vi "Simulated Starter Kit 2.0 Roaming.vi"() -> ()   [LabVIEW 2017]
doc: "This VI demonstrates how to control a simulated Robotics Starter Kit 2.0 robot. With a few modifications, you can deploy this VI to the Single-Board RIO 9632 on a real robot, and it runs on the real-time controller. For more information about how to modify this VI so you can deploy it to real hardware, refer to the <B>Robotics Module>>Simulating Mobile Robots</B> book on the <B>Contents</B> tab of the LabVIEW Help."
uses:
  <vilib>/Platform/TimedLoop/XDataNode/timing_clust.ctl
  <vilib>/Platform/TimedLoop/XDataNode/nitl_modes.ctl
  <vilib>/Platform/TimedLoop/XDataNode/wakeup.ctl
  <vilib>/robotics/Simulator/Engine/ctl/Step Mode.ctl
  <vilib>/robotics/Steering/Differential Steering Frame/NI_Robotics_Differential Steering Frame.lvclass
  E:/Labview/NI/LabVIEW 2017/vi.lib/robotics/Steering/Steering Frame/NI_Robotics_Steering Frame.lvclass
  <vilib>/robotics/Starter Kit/2.0/Sim Host Interface/NI_Robotics_Starter Kit Host_Sim_2.0.lvclass
  E:/Labview/NI/LabVIEW 2017/vi.lib/robotics/Starter Kit/Host Interface/NI_Robotics_Starter Kit Host.lvclass
  <vilib>/robotics/Simulator/Interface/Simulator References/Get Robot Body Reference.vi
  <vilib>/robotics/Steering/Steering Frame/Apply Steering Frame Velocity to Motors.vi
  <vilib>/Platform/TimedLoop/XDataNode/XDataNode.xnode
  <vilib>/Platform/TimedLoop/XDataNode/XDNodeRunTimeDep.lvlib
  <vilib>/robotics/Steering/Steering Frame/NI_Robotics_Steering Frame.lvclass
  <vilib>/robotics/Starter Kit/Host Interface/NI_Robotics_Starter Kit Host.lvclass
  <vilib>/robotics/Starter Kit/2.0/NI_Robotics_Starter Kit Host_2.0.lvlib
  <vilib>/robotics/Simulator/NI_Robotics_Simulator.lvlib
  <resource>/objmgr/LVODE.rc
  E:/Labview/NI/LabVIEW 2017/vi.lib/robotics/Steering/Special Steering Frame/NI_Robotics_Special Steering Frame.lvclass
panel:
  out "pausing":dbl
  out "v":dbl[](array[numeric])
  out "mov":dbl
  out "pause_time":dbl
  out "st_time":dbl
  out "cord":sgl[](array[numeric])
  out "dir":dbl[](array[numeric])
  out "ind":dbl
  out "Time":i64
  out "appended path":path
  out "Position":sgl[](array[numeric])
  out "Robot Position":cluster{sgl[], sgl[]}[](graph)
  in  "stop 2":bool
  out "Path 2":dbl[][](array[numeric])
  out "Path":dbl[][](array[numeric])
  out "Intensity Graph":dbl[][](graph)
  in  "stop":bool
  # "This VI demonstrates how to control a simulated Robotics Starter Kit 2.0 robot.\n\nRun this VI to launch the simulation.  The simulated environment is displayed in a separate window.  The graph displays the range data acquired by the simulated ultrasonic sensor on the robot.  Click the STOP button to end the simulation."
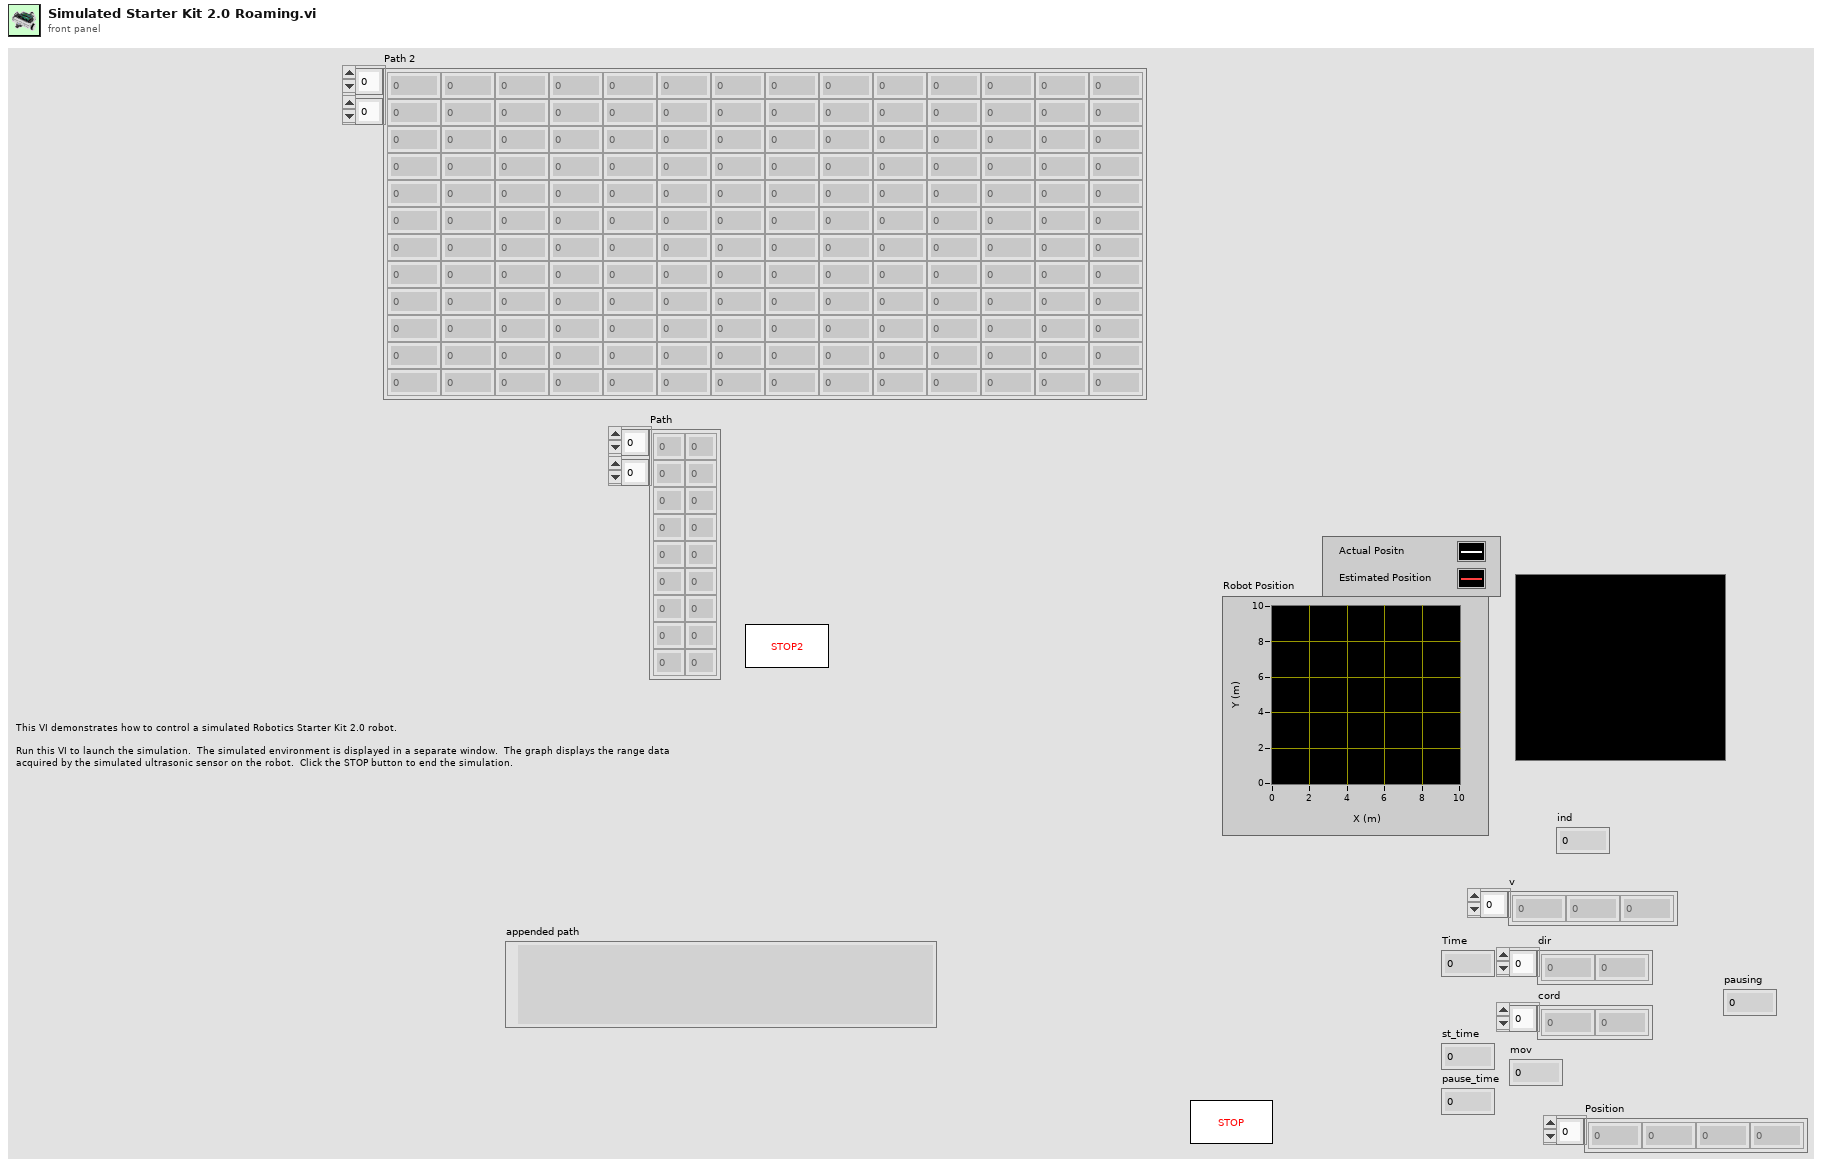
[diagram p1: front panel]
types:
  T1 = typedef "NI_Robotics_Simulator.lvlib/Step Mode.ctl" = u16
  T2 = typedef "XDNodeRunTimeDep.lvlib/timing_clust.ctl" = cluster{"Expected End [f-1]":u64, "Actual End [f-1]":u64, "Finished Late? [f-1]":bool, "Expected End [i-1]":u64, "Actual End [i-1]":u64, "Finished Late? [i-1]":bool, "Expected Start [i]":u64, "Actual Start [i]":u64, "Expected Start [f]":u64, "Actual Start [f]":u64, "Source Name":string, "Structure Name":string, "Period":i64, "Deadline":i64, "Offset":i64, "Start":i64, "Priority":i32, "Timeout":i32, "Mode":T3, "Wakeup Reason":T4, "Error":errorcluster, "Source Type":string, "Secondary Source Type":string, "Global End Time":u64, "Global Start Time":u64, "Frame Duration":u64, "Iteration Duration":u64, "Assigned CPU":i32, "I/O Scan Engine Mode":u32}
  T3 = typedef "XDNodeRunTimeDep.lvlib/nitl_modes.ctl" = enum32{"No Change", "Process missed periods, maintain original phase", "Discard missed periods, maintain original phase", "Process missed periods, ignore original phase", "Discard missed periods, ignore original phase"}
  T4 = typedef "XDNodeRunTimeDep.lvlib/wakeup.ctl" = enum32{"Normal", "Aborted", "Asynchronous wakeup", "Timing source error", "Timed loop error", "Timeout"}
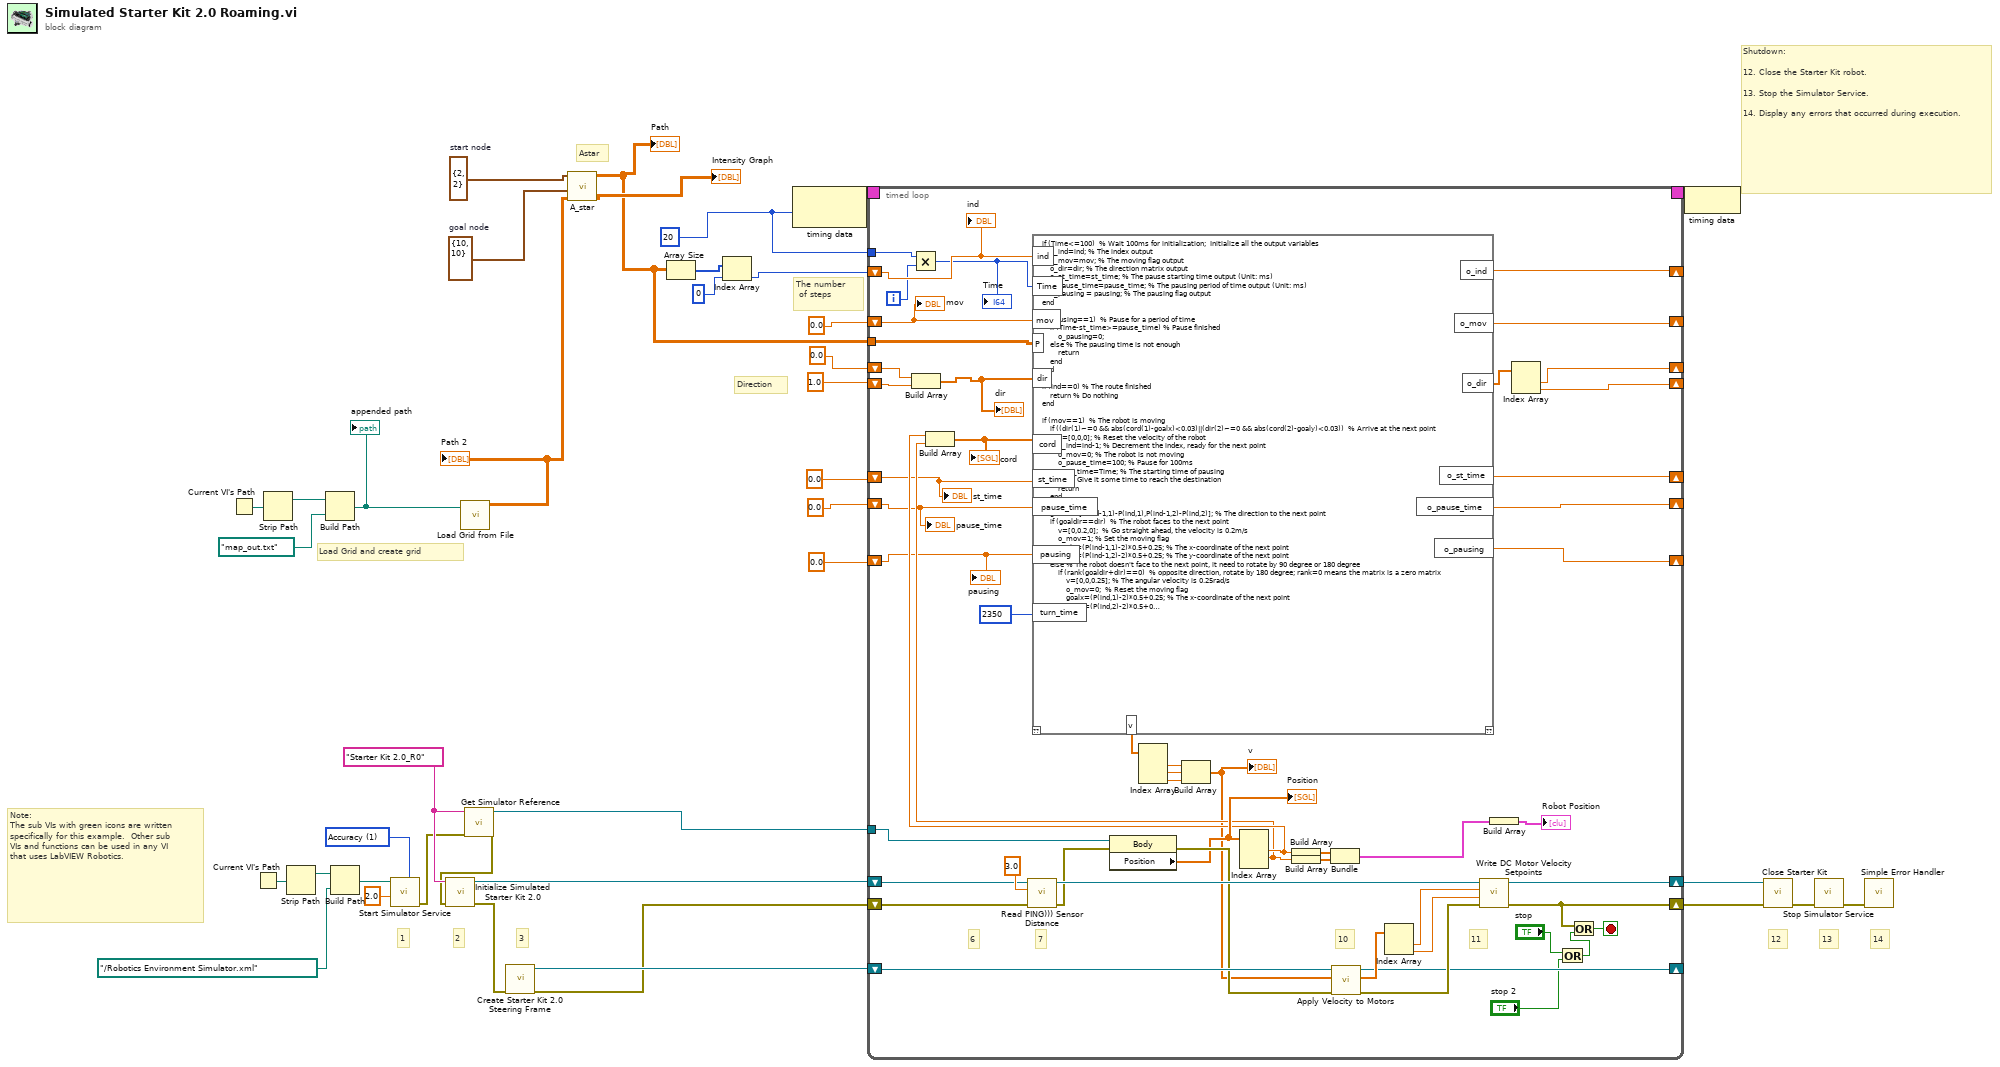
[diagram p0: block diagram]
diagram:
  w2 = cluster{"X":i32, "Y":i32} {"X"=10, "Y"=10}  # goal node
  w3 = cluster{"X":i32, "Y":i32} {"X"=2, "Y"=2}  # start node
  w24 = T1 1 items=["Performance", "Accuracy"] ("step mode")
  w19 = "Starter Kit 2.0_R0" ("robot ID")
  w13 = i64 20 ("Period")
  # "The number\n of steps"
  # "Direction"
  # "Astar"
  # "Load Grid and create grid"
  # "14"
  # "13"
  # "12"
  # "1"
  # "Shutdown:\n\n12. Close the Starter Kit robot.\n\n13. Stop the Simulator Service.\n\n14. Display any errors that occurred during execution."
  # "Note:\nThe sub VIs with green icons are written specifically for this example.  Other sub VIs and functions can be used in any VI that uses LabVIEW Robotics."
  # "2"
  # "3"
  n1 = Current VI's Path() -> (path=w23:path)
  n2 = Current VI's Path() -> (path=w38:path)
  n3 = Strip Path(path=w23) -> (stripped path=w22:path)  [unwired: 1 out]
  n4 = Strip Path(path=w38) -> (stripped path=w39:path)  [unwired: 1 out]
  n5 = Build Path(base path=w22, name or relative path=path "map_out.txt" ("stripped path")) -> (appended path=w20:path)
  "appended path" <- w20
  n6 = Build Path(base path=w39, name or relative path=path "../Robotics Environment Simulator.xml" ("Simulation Manifest File")) -> (appended path=w28:path)
  n7 = call <vilib>:"Start Simulator Service.vi"("step mode"=w24, "step size (ms)"=2.0, "manifest file"=w28) -> ("error out"=w18:errorcluster)  [unwired: 8 in]
  n8 = call "Load Grid from File.vi"("file path"=w20) -> ("occupancy grid"=w1:dbl[][])  [unwired: 8 in, 2 out]
  "Path 2" <- w1
  n9 = call-poly <vilib>:"Get Simulator Reference.vi"("error in (no error)"=w18, "robot ID"=w19) -> ("error out"=w17:errorcluster, "robot body ref"=w16:refnum<k20>)  [unwired: 8 in]
  n10 = call <vilib>:"Initialize Simulated Starter Kit 2.0.vi"("error in (no error)"=w17, "robot ID"=w19) -> ("error out"=w33:errorcluster, "simulated starter kit host 2.0 out"=w34:refnum<class "NI_Robotics_Starter Kit Host_Sim_2.0.lvclass">)  [unwired: 8 in]
  n11 = call <vilib>:"Create Starter Kit 2.0 Steering Frame.vi"("error in (no error)"=w33) -> ("error out"=w30:errorcluster, "starter kit differential steering frame"=w35:refnum<class "NI_Robotics_Differential Steering Frame.lvclass">)  [unwired: 9 in]
  n12 = call "A_star.vi"("Map"=w1, "Ed"=w2, "St"=w3) -> ("Map_out"=→"Intensity Graph":dbl[][], "Path"=w4:dbl[][])  [unwired: 7 in]
  "Path" <- w4
  n13 = Array Size(array=w4) -> (size(s)=w15:i32[])
  n14 = Index Array(array=w15, index=0 ("Period")) -> (element=w6:i32)
  n15 = node-c288(w13) -> (w37:T2)
  n16 = timed-loop {
    shift-right: [w86] -> w32
    shift-left: w34 -> [w81]
    shift-right: [w85] -> w31
    shift-left: w30 -> [w80]
    shift-right: [w88] -> _
    shift-left: w35 -> [w89]
    timing: w37 -> [_]
    timing-out: [_] -> w36
    shift-right: [w67] -> _
    shift-left: w6 -> [w68]
    tunnel: w16 -> [w75]
    tunnel: w13 -> [w62]
    tunnel: w4 -> [w55]
    shift-right: [w53] -> _
    shift-left: 0.0 ("Period") -> [w54]
    shift-right: [w51] -> _
    shift-left: 0.0 ("Period") -> [w52]
    shift-right: [w49] -> _
    shift-left: 0.0 ("Period") -> [w50]
    shift-right: [w44] -> _
    shift-left: 0.0 ("Period") -> [w47]
    shift-right: [w43] -> _
    shift-left: 1.0 ("Period") -> [w48]
    shift-right: [w41] -> _
    shift-left: 0.0 ("Period") -> [w42]
    i -> [w63]
    stop <- w87 stop-if-true
    # "7"
    # "6"
    # "11"
    # "10"
    n17 = Multiply(x=w62, y=w63) -> (x*y=w61:i64)
    "Time" <- w61
    n18 = Build Array(w47, w48) -> (w46:dbl[])
    "dir" <- w46
    n19 = call <vilib>:"Read PING))) Sensor Distance.vi"("error in (no error)"=w80, "default distance (NaN)"=3.0, "starter kit host in"=w81) -> ("error out"=w74:errorcluster, "starter kit host out"=w84:refnum<class "NI_Robotics_Starter Kit Host_Sim_2.0.lvclass">)  [unwired: 5 in, 2 out]
    n20 = property class="Body"(reference=w75, error in=w74) -> (error out=w73:errorcluster, "Position"=w70:sgl[])  [unwired: 1 out]
    "Position" <- w70
    n21 = Index Array(array=w70) -> (element #1=w66:sgl, element #2=w65:sgl)  [unwired: 3 in, 1 out]
    n22 = Build Array(w66, w65) -> (w64:sgl[])
    "cord" <- w64
    n23 = script code="if (Time<=100)  % Wait 100ms for initialization;  Initialize all the output variables\n    o_ind=ind; % The index output\n    o_mov=mov; % The moving flag output \n    o_dir=dir; % The direction matrix output\n    o_st_time=st_time; % The pause starting time output (Unit: ms)\n    o_pause_time=pause_time; % The pausing period of time output (Unit: ms)\n    o_pausing = pausing; % The pausing flag output\nend\n\nif (pausing==1)  % Pause for a period of time\n    if (Time-st_time>=pause_time) % Pause finished\n        o_pausing=0; \n    else % The pausing time is not enough\n        return \n    end\nend\n\nif (ind==0) % The route finished\n    return % Do nothing\nend\n\nif (mov==1)  % The robot is moving\n    if ((dir(1)~=0 && abs(cord(1)-goalx)<0.03)||(dir(2)~=0 && abs(cord(2)-goaly)<0.03))  % Arrive at the next point\n        v=[0,0,0]; % Reset the velocity of the robot\n        o_ind=ind-1; % Decrement the index, ready for the next point\n        o_mov=0; % The robot is not moving\n        o_pause_time=100; % Pause for 100ms\n        o_st_time=Time; % The starting time of pausing\n    else  % Give it some time to reach the destination\n        return\n    end\nelse\n    goaldir=[P(ind-1,1)-P(ind,1),P(ind-1,2)-P(ind,2)]; % The direction to the next point\n    if (goaldir==dir)  % The robot faces to the next point\n        v=[0,0.2,0];  % Go straight ahead, the velocity is 0.2m/s\n        o_mov=1; % Set the moving flag\n        goalx=(P(ind-1,1)-2)*0.5+0.25; % The x-coordinate of the next point\n        goaly=(P(ind-1,2)-2)*0.5+0.25; % The y-coordinate of the next point\n    else % The robot doesn't face to the next point, it need to rotate by 90 degree or 180 degree\n        if (rank(goaldir+dir)==0)  % opposite direction, rotate by 180 degree; rank=0 means the matrix is a zero matrix\n            v=[0,0,0.25]; % The angular velocity is 0.25rad/s\n            o_mov=0;  % Reset the moving flag\n            goalx=(P(ind,1)-2)*0.5+0.25; % The x-coordinate of the next point\n            goaly=(P(ind,2)-2)*0.5+0.25; % The y-coordinate of the next point\n            o_dir=goaldir; % The direction of the robot is set to the direction to the next point\n            o_pause_time=4700; % The rotating time is 9640ms\n            o_pausing=1; % Set the pausing flag\n            o_st_time=Time;  % Mark the starting time\n        else  % Rotate by 90 degree\n            gd_a=goaldir(1)*10+goaldir(2);\n            d_a=dir(1)*10+dir(2);\n            A_a=[1,10,-1,-10,1]; % Standing for 4 directions\n            ccw=0; % Counter clockwise or not\n            for i=1:4\n                if (gd_a==A_a(i)&&d_a==A_a(i+1)) % Counter clockwise\n                    ccw=1; \n                    break;\n                end\n                if (gd_a==A_a(i+1)&&d_a==A_a(i)) % Clockwise\n                    ccw=0; \n                    break;\n                end\n            end\n            v=[0,0,-0.3+ccw*0.6]; % The angular velocity is 0.3rad/s\n            o_mov=0; % Reset the moving flag\n            o_dir=goaldir;  % Mark the direction\n            goalx=(P(ind,1)-2)*0.5+0.25; % The x-coordinate of the next point\n            goaly=(P(ind,2)-2)*0.5+0.25; % The y-coordinate of the next point\n            o_pausing=1; % Set the pausing flag\n            o_pause_time=turn_time; % The rotating time period\n            o_st_time=Time; % Mark the starting time\n        end\n    end\nend"("ind"=w68, "mov"=w50, "cord"=w64, "dir"=w46, "Time"=w61, "P"=w55, "st_time"=w54, "pause_time"=w52, "pausing"=w42, "turn_time"=2350) -> ("o_ind"=w67:dbl, "o_dir"=w45:dbl[], "o_mov"=w49:dbl, "v"=w60:dbl[], "o_st_time"=w53:dbl, "o_pause_time"=w51:dbl, "o_pausing"=w41:dbl)  [unwired: 1 in, 1 out]
    n24 = Index Array(array=w60) -> (element #1=w59:dbl, element #2=w58:dbl, element #3=w57:dbl)  [unwired: 3 in]
    n25 = Build Array(w59, w58, w57) -> (w56:dbl[])
    "v" <- w56
    n26 = Build Array(w66) -> (w71:sgl[])
    n27 = Build Array(w65) -> (w72:sgl[])
    n28 = Bundle(w71, w72) -> (w69:cluster{sgl[], sgl[]})  [unwired: 1 in]
    n29 = call-poly <vilib>:"Apply Velocity to Motors.vi"("error in (no error)"=w73, "steering frame velocity"=w56, "steering frame in"=w89) -> ("error out"=w91:errorcluster, "ccw motor velocity setpoints"=w92:dbl[], "steering frame out"=w88:refnum<class "NI_Robotics_Differential Steering Frame.lvclass">)  [unwired: 4 in, 2 out]
    n30 = Index Array(array=w92) -> (element #1=w83:dbl, element #2=w82:dbl)  [unwired: 2 in]
    n31 = call <vilib>:"Write DC Motor Velocity Setpoints.vi"("error in (no error)"=w91, "right motor ccw velocity (rad/s)"=w82, "left motor ccw velocity (rad/s)"=w83, "starter kit host in"=w84) -> ("error out"=w85:errorcluster, "starter kit host out"=w86:refnum<class "NI_Robotics_Starter Kit Host_Sim_2.0.lvclass">)  [unwired: 6 in]
    n32 = Build Array(w69) -> (→"Robot Position":cluster{sgl[], sgl[]}[])
    n33 = Index Array(array=w45) -> (element #1=w44:dbl, element #2=w43:dbl)  [unwired: 2 in]
    n34 = Or(x="stop", y="stop 2") -> (x .or. y?=w77:bool)
    n35 = Or(x=w85, y=w77) -> (x .or. y?=w87:bool)
    "ind" <- w68
    "st_time" <- w54
    "pause_time" <- w52
    "mov" <- w50
    "pausing" <- w42
  }
  n36 = node-c288(w36) -> ()
  n37 = call-dynamic "Close Starter Kit.vi"("error in (no error)"=w31, "starter kit host in"=w32) -> ("error out"=w26:errorcluster)  [unwired: 9 in]
  n38 = call <vilib>:"Stop Simulator Service.vi"("error in (no error)"=w26) -> ("error out"=w25:errorcluster)  [unwired: 10 in]
  n39 = call <vilib>:"Simple Error Handler.vi"("error in (no error)"=w25) -> ()  [unwired: 4 in, 5 out]
